vi "SinAtan2.vi"(10 "X":dbl, 11 "Y":dbl) -> (2 "cos(atan2(x,y))":dbl, 3 "sin(atan2(x,y))":dbl)   [LabVIEW 2012]
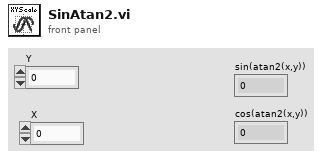
[diagram p1: front panel]
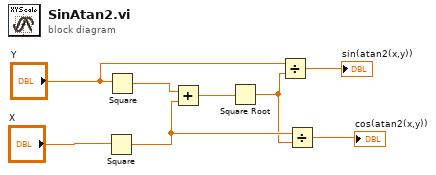
[diagram p0: block diagram]
diagram:
  n1 = Square(x="X") -> (x^2=w3:dbl)
  n2 = Square(x="Y") -> (x^2=w8:dbl)
  n3 = Add(x=w8, y=w3) -> (x+y=w7:dbl)
  n4 = Square Root(x=w7) -> (sqrt(x)=w2:dbl)
  n5 = Divide(x="Y", y=w2) -> (x/y=→"sin(atan2(x,y))":dbl)
  n6 = Divide(x=w3, y=w2) -> (x/y=→"cos(atan2(x,y))":dbl)
